vi "Drive_Queue.vi"   [LabVIEW 2009, in "Drive.lvlib"]
uses:
  Drive.lvlib
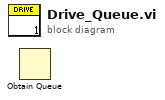
[diagram p0: block diagram]
diagram:
  n1 = Obtain Queue() -> ()  [unwired: 5 in, 3 out]
